vi "Clear All Discretes.vi"(8 "error in":errorcluster, 11 "ProXR_IO in":refnum<class "ProXR.lvclass">) -> (0 "error out":errorcluster, 3 "ProXR_IO out":refnum<class "ProXR.lvclass">)   [LabVIEW 2019, in "ProXR.lvlib" / "ProXR.lvclass"]
uses:
  Library/ProXR.lvclass
  builds/Instruments/DIG_IO.lvlibp/Library/DIG_IO.lvclass
panel:
  out "Response":u8[](array[numeric])
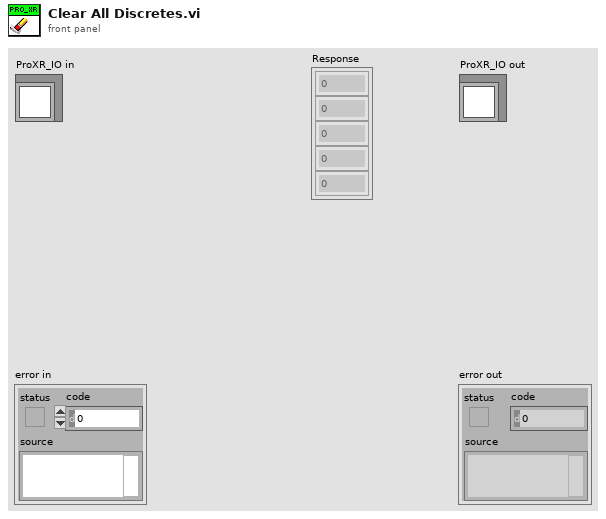
[diagram p1: front panel]
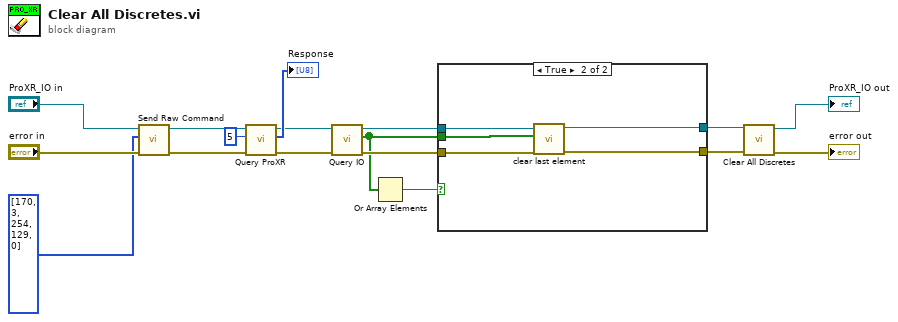
[diagram p0: block diagram]
diagram:
  n1 = call "Send Raw Command.vi"("error in"="error in", "Raw Command"=u8[] [170, 3, 254, 129, 0], "ProXR_IO in"="ProXR_IO in") -> ("error out"=w13:errorcluster, "ProXR_IO out"=w14:refnum<class "ProXR.lvclass">)  [unwired: 7 in]
  n2 = call "Query ProXR.vi"("error in"=w13, "Bytes to Read"=u32 5, "ProXR_IO in"=w14) -> ("error out"=w7:errorcluster, "Response"=→"Response":u8[], "ProXR_IO out"=w8:refnum<class "ProXR.lvclass">)  [unwired: 6 in]
  n3 = call-dynamic "Query IO.vi"("error in"=w7, "ProXR in"=w8) -> ("error out"=w4:errorcluster, "Boolean Array"=w3:bool[], "ProXR out"=w5:refnum<class "ProXR.lvclass">)  [unwired: 6 in, 1 out]
  n4 = Or Array Elements(Boolean array=w3) -> (logical OR=w6:bool)
  n5 = case shown="True" w6 {
    tunnel: w5 -> [w19 w23]
    tunnel: w4 -> [w18 w24]
    tunnel: w3 -> [_ w22]
    tunnel: [w19 w21] -> w2
    tunnel: [w18 w20] -> w1
    frame False {
    }
    frame True {
      n6 = call "clear last element.vi"("error in"=w24, "Boolean Array"=w22, "ProXR in"=w23) -> ("error out"=w20:errorcluster, "ProXR out"=w21:refnum<class "ProXR.lvclass">)  [unwired: 7 in]
    }
  }
  n7 = call-parent "Clear All Discretes.vi"("error in"=w1, "DIG_IO in"=w2) -> ("error out"=→"error out":errorcluster, "DIG_IO out"=→"ProXR_IO out":refnum<class "ProXR.lvclass">)  [unwired: 8 in]
